vi "Organize Scouting Data.vi"() -> ()   [LabVIEW 2015]
uses:
  <vilib>/Utility/sysdir.llb/System Directory Type.ctl
panel:
  out "array averaged":string[][](array[string])
  out "array":string[][](array[string])
  out "reversed array":T1(array[cluster])
  in  "input cluster":T2
  out "output cluster":T2
  in  "Sort By":u16(ring) items=["Team Number", "Rating", "Number of High Goals", "Number of Low Goals"]
  in  "array type (2D Dbl)":string[][](array[string])
  # "Team Number"
  # "Lift Gate"
  # "Teeter Totter"
  # "Moat"
  # "Rampart"
  # "Drawbridge"
  # "Sally Port"
  # "Rock Wall"
  # "Rough Terrain"
  # "Low Bar"
  # "Auto High Goal"
  # "Auto Low Goal"
  # "Scale"
  # "High Goals"
  # "Low Goal"
  # "Autonomous"
  # "Up to Defense"
  # "Rating"
  # "Comment"
  # "Team Number"
  # "Lift Gate"
  # "Teeter Totter"
  # "Moat"
  # "Rampart"
  # "Drawbridge"
  # "Sally Port"
  # "Rock Wall"
  # "Rough Terrain"
  # "Low Bar"
  # "Auto High Goal"
  # "Auto Low Goal"
  # "Scale"
  # "High Goals"
  # "Low Goal"
  # "Autonomous"
  # "Up to Defense"
  # "Rating"
  # "Comment"
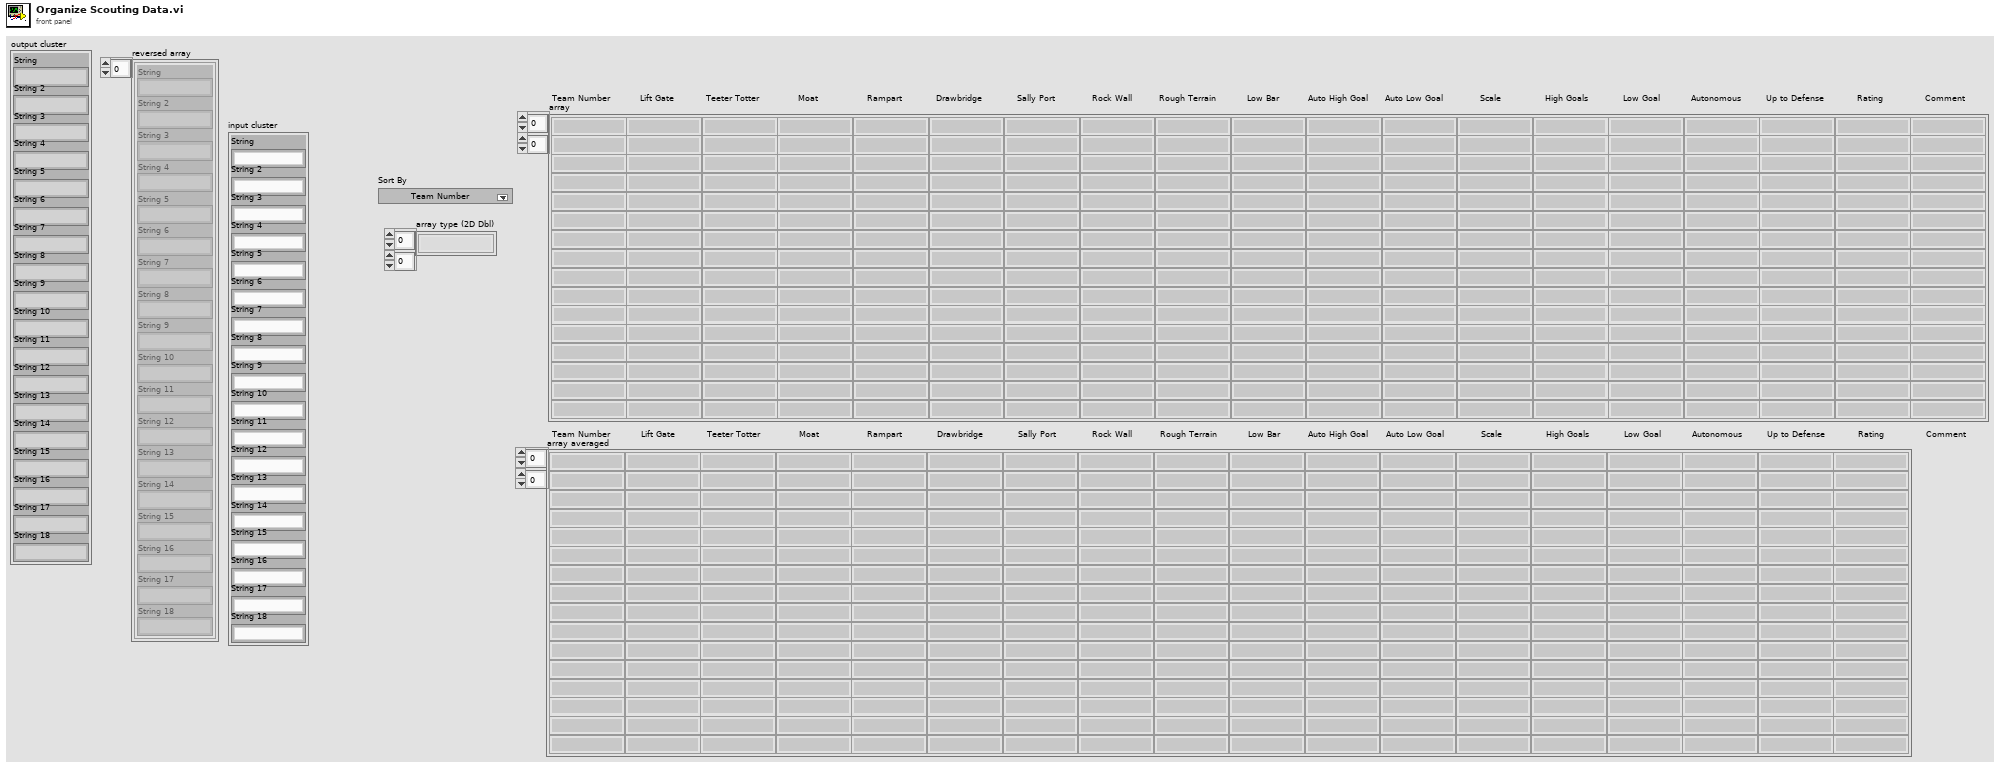
[diagram p1: front panel]
types:
  T1 = cluster{"String":string, "String 2":string, "String 3":string, "String 4":string, "String 5":string, "String 6":string, "String 7":string, "String 8":string, "String 9":string, "String 10":string, "String 11":string, "String 12":string, "String 13":string, "String 14":string, "String 15":string, "String 16":string, "String 17":string, "String 18":string}[]
  T2 = cluster{"String":string, "String 2":string, "String 3":string, "String 4":string, "String 5":string, "String 6":string, "String 7":string, "String 8":string, "String 9":string, "String 10":string, "String 11":string, "String 12":string, "String 13":string, "String 14":string, "String 15":string, "String 16":string, "String 17":string, "String 18":string}
  T3 = typedef "System Directory Type.ctl" = i32
  T4 = enum16{"open", "replace", "create", "open or create", "replace or create", "replace or create with confirmation"}
  T5 = cluster{string, string, string, string, string, string, string, string, string, string, string, string, string, string, string, string, string, string, string}[]
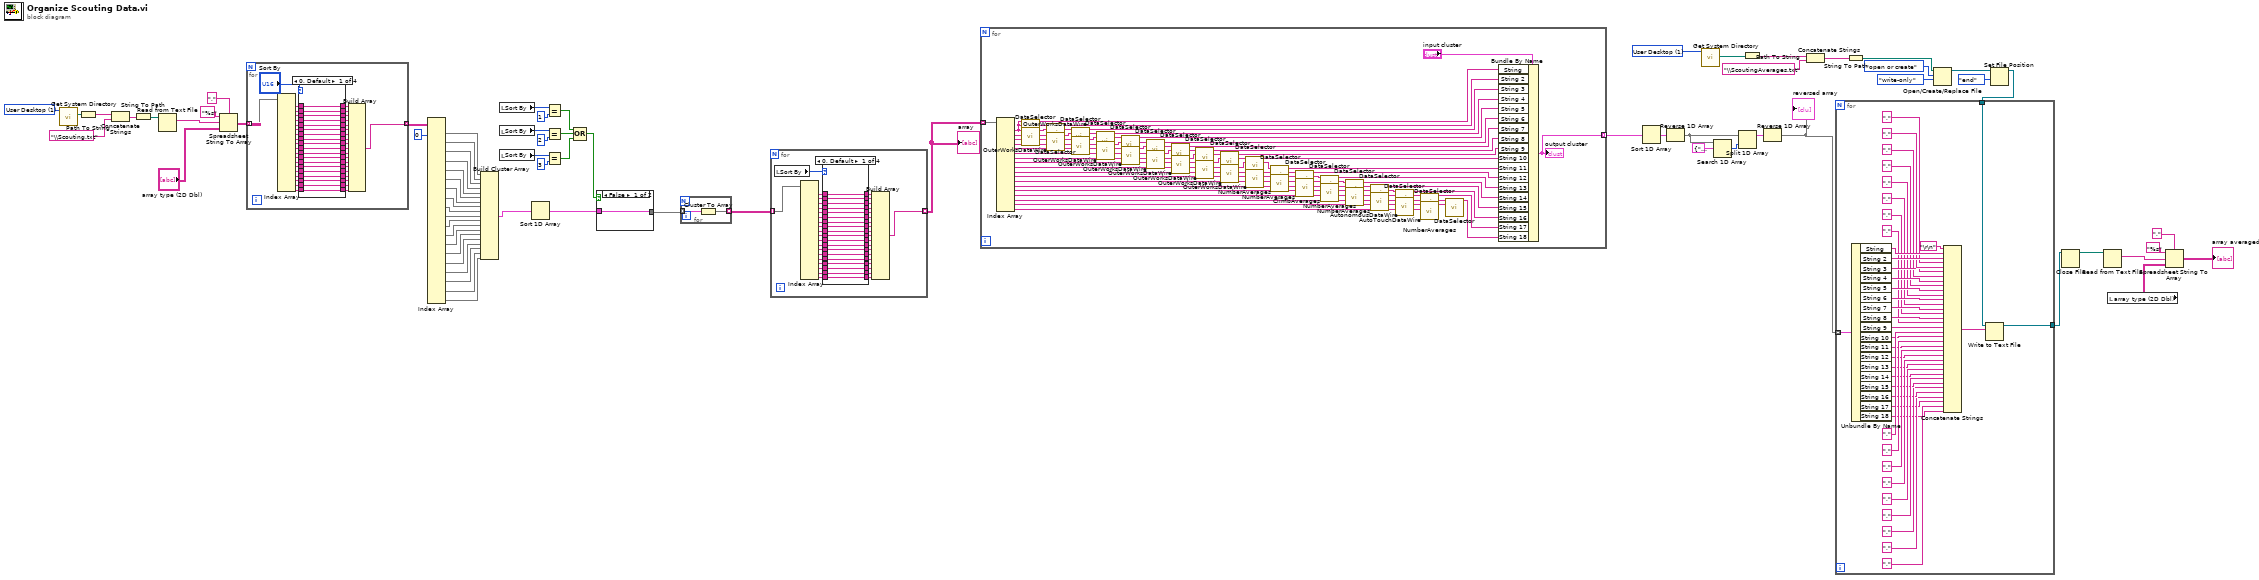
[diagram p0: block diagram]
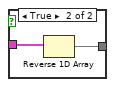
[diagram p5: hidden frame]
diagram:
  w15 = T3 1 items=["User Home"=0, "User Desktop"=1, "User Documents"=2, "User Application Data"=3, "User Preferences"=4, "User Temporary"=5, "Public Documents"=6, "Public Application Data"=7, "Public Preferences"=8, "Public Cache"=13, "System Core Libraries"=9, "System Installed Libraries"=10, "Application Files"=11, "Boot Volume Root"=12] ("system directory type")
  w68 = T3 1 items=["User Home"=0, "User Desktop"=1, "User Documents"=2, "User Application Data"=3, "User Preferences"=4, "User Temporary"=5, "Public Documents"=6, "Public Application Data"=7, "Public Preferences"=8, "Public Cache"=13, "System Core Libraries"=9, "System Installed Libraries"=10, "Application Files"=11, "Boot Volume Root"=12] ("system directory type")
  n1 = call <vilib>:"Get System Directory.vi"("system directory type"=w68) -> ("system directory"=w69:path)  [unwired: 10 in]
  n2 = Path To String(path=w69) -> (string=w70:string)
  n3 = Concatenate Strings(w70, "\\Scouting.txt" ("string")) -> (w72:string)
  n4 = String To Path(string=w72) -> (path=w67:path)
  n5 = Read from Text File(file (use dialog)=w67) -> (text=w64:string)  [unwired: 3 in, 3 out]
  n6 = Spreadsheet String To Array(delimiter (Tab)=",", format string="%s", spreadsheet string=w64, array type (2D Dbl)="array type (2D Dbl)") -> (array=w56:string[][])
  n7 = for {
    tunnel: w56 -> [w113] mode=indexing
    tunnel: [w76] -> w35 mode=indexing
    n8 = Index Array(array=w113) -> (element #1=w111:string, element #2=w109:string, element #3=w108:string, element #4=w105:string, element #5=w103:string, element #6=w101:string, element #7=w99:string, element #8=w97:string, element #9=w95:string, element #10=w93:string, element #11=w91:string, element #12=w89:string, element #13=w87:string, element #14=w85:string, element #15=w83:string, element #16=w81:string, element #17=w79:string, element #18=w77:string, element #19=w73:string)  [unwired: 19 in]
    n9 = case shown="0, Default" "Sort By" {
      tunnel: [w132 w150 w170 w172] -> w112
      tunnel: w111 -> [w132 w151 w169 w173]
      tunnel: [w131 w149 w168 w189] -> w110
      tunnel: w109 -> [w131 w149 w168 w189]
      tunnel: [w130 w148 w167 w188] -> w107
      tunnel: w108 -> [w130 w148 w167 w188]
      tunnel: [w129 w147 w166 w187] -> w106
      tunnel: w105 -> [w129 w147 w166 w187]
      tunnel: [w128 w146 w165 w186] -> w104
      tunnel: w103 -> [w128 w146 w165 w186]
      tunnel: [w127 w145 w164 w185] -> w102
      tunnel: w101 -> [w127 w145 w164 w185]
      tunnel: [w126 w144 w163 w184] -> w100
      tunnel: w99 -> [w126 w144 w163 w184]
      tunnel: [w125 w143 w162 w183] -> w98
      tunnel: w97 -> [w125 w143 w162 w183]
      tunnel: [w124 w142 w161 w182] -> w96
      tunnel: w95 -> [w124 w142 w161 w182]
      tunnel: [w123 w141 w160 w181] -> w94
      tunnel: w93 -> [w123 w141 w160 w181]
      tunnel: [w122 w140 w159 w180] -> w92
      tunnel: w91 -> [w122 w140 w159 w180]
      tunnel: [w121 w139 w158 w179] -> w90
      tunnel: w89 -> [w121 w139 w158 w179]
      tunnel: [w120 w138 w157 w178] -> w88
      tunnel: w87 -> [w120 w138 w157 w178]
      tunnel: [w119 w137 w169 w171] -> w86
      tunnel: w85 -> [w119 w137 w170 w171]
      tunnel: [w118 w136 w156 w173] -> w84
      tunnel: w83 -> [w118 w136 w156 w172]
      tunnel: [w117 w135 w155 w177] -> w82
      tunnel: w81 -> [w117 w135 w155 w177]
      tunnel: [w116 w134 w154 w176] -> w80
      tunnel: w79 -> [w116 w134 w154 w176]
      tunnel: [w115 w151 w153 w175] -> w78
      tunnel: w77 -> [w115 w150 w153 w175]
      tunnel: [w114 w133 w152 w174] -> w74
      tunnel: w73 -> [w114 w133 w152 w174]
      frame 0, Default {
      }
      frame 1 {
      }
      frame 2 {
      }
      frame 3 {
      }
    }
    n10 = Build Array(w112, w110, w107, w106, w104, w102, w100, w98, w96, w94, w92, w90, w88, w86, w84, w82, w80, w78, w74) -> (w76:string[])
  }
  n11 = Index Array(array=w35, index (col) #1=0 ("disabled index (col)")) -> (element #1=w55:string[], element #2=w54:string[], element #3=w53:string[], element #4=w52:string[], element #5=w51:string[], element #6=w50:string[], element #7=w49:string[], element #8=w48:string[], element #9=w47:string[], element #10=w46:string[], element #11=w45:string[], element #12=w44:string[], element #13=w43:string[], element #14=w42:string[], element #15=w41:string[], element #16=w40:string[], element #17=w39:string[], element #18=w38:string[], element #19=w36:string[])  [unwired: 37 in]
  n12 = Build Cluster Array ("Index & Bundle Cluster Array")(w55, w54, w53, w52, w51, w50, w49, w48, w47, w46, w45, w44, w43, w42, w41, w40, w39, w38, w36) -> (w37:T5)
  n13 = local read "Sort By"() -> (w32:u16)
  n14 = local read "Sort By"() -> (w29:u16)
  n15 = local read "Sort By"() -> (w28:u16)
  n16 = Sort 1D Array(array=w37) -> (sorted array=w34:T5)
  n17 = Equal?(x=w32, y=u16 1) -> (x = y?=w26:bool)
  n18 = Equal?(x=w29, y=u16 2) -> (x = y?=w25:bool)
  n19 = Equal?(x=w28, y=u16 3) -> (x = y?=w24:bool)
  n20 = Compound Arithmetic op=OR(w26, w25, w24) -> (w23:bool)
  n21 = case shown="False" w23 {
    tunnel: w34 -> [w190 w192]
    tunnel: [w190 w191] -> w33
    frame False {
    }
    frame True {
      n22 = Reverse 1D Array(array=w192) -> (reversed array=w191:T5)
    }
  }
  n23 = for {
    tunnel: w33 -> [w193] mode=indexing
    tunnel: [w194] -> w22 mode=indexing
    n24 = Cluster To Array(cluster=w193) -> (array=w194:string[])
  }
  n25 = for {
    tunnel: w22 -> [w235] mode=indexing
    tunnel: [w198] -> w20 mode=indexing
    n26 = local read "Sort By"() -> (w195:u16)
    n27 = Index Array(array=w235) -> (element #1=w233:string, element #2=w231:string, element #3=w230:string, element #4=w227:string, element #5=w225:string, element #6=w223:string, element #7=w221:string, element #8=w219:string, element #9=w217:string, element #10=w215:string, element #11=w213:string, element #12=w211:string, element #13=w209:string, element #14=w207:string, element #15=w205:string, element #16=w203:string, element #17=w201:string, element #18=w199:string, element #19=w196:string)  [unwired: 19 in]
    n28 = case shown="0, Default" w195 {
      tunnel: [w254 w272 w292 w294] -> w234
      tunnel: w233 -> [w254 w273 w291 w295]
      tunnel: [w253 w271 w290 w311] -> w232
      tunnel: w231 -> [w253 w271 w290 w311]
      tunnel: [w252 w270 w289 w310] -> w229
      tunnel: w230 -> [w252 w270 w289 w310]
      tunnel: [w251 w269 w288 w309] -> w228
      tunnel: w227 -> [w251 w269 w288 w309]
      tunnel: [w250 w268 w287 w308] -> w226
      tunnel: w225 -> [w250 w268 w287 w308]
      tunnel: [w249 w267 w286 w307] -> w224
      tunnel: w223 -> [w249 w267 w286 w307]
      tunnel: [w248 w266 w285 w306] -> w222
      tunnel: w221 -> [w248 w266 w285 w306]
      tunnel: [w247 w265 w284 w305] -> w220
      tunnel: w219 -> [w247 w265 w284 w305]
      tunnel: [w246 w264 w283 w304] -> w218
      tunnel: w217 -> [w246 w264 w283 w304]
      tunnel: [w245 w263 w282 w303] -> w216
      tunnel: w215 -> [w245 w263 w282 w303]
      tunnel: [w244 w262 w281 w302] -> w214
      tunnel: w213 -> [w244 w262 w281 w302]
      tunnel: [w243 w261 w280 w301] -> w212
      tunnel: w211 -> [w243 w261 w280 w301]
      tunnel: [w242 w260 w279 w300] -> w210
      tunnel: w209 -> [w242 w260 w279 w300]
      tunnel: [w241 w259 w291 w293] -> w208
      tunnel: w207 -> [w241 w259 w292 w293]
      tunnel: [w240 w258 w278 w295] -> w206
      tunnel: w205 -> [w240 w258 w278 w294]
      tunnel: [w239 w257 w277 w299] -> w204
      tunnel: w203 -> [w239 w257 w277 w299]
      tunnel: [w238 w256 w276 w298] -> w202
      tunnel: w201 -> [w238 w256 w276 w298]
      tunnel: [w237 w273 w275 w297] -> w200
      tunnel: w199 -> [w237 w272 w275 w297]
      tunnel: [w236 w255 w274 w296] -> w197
      tunnel: w196 -> [w236 w255 w274 w296]
      frame 0, Default {
      }
      frame 1 {
      }
      frame 2 {
      }
      frame 3 {
      }
    }
    n29 = Build Array(w234, w232, w229, w228, w226, w224, w222, w220, w218, w216, w214, w212, w210, w208, w206, w204, w202, w200, w197) -> (w198:string[])
  }
  "array" <- w20
  n30 = for {
    tunnel: w20 -> [w400] mode=indexing
    tunnel: [w399] -> w62 mode=indexing
    n31 = Index Array(array=w400) -> (element #1=w337:string, element #2=w336:string, element #3=w335:string, element #4=w334:string, element #5=w333:string, element #6=w332:string, element #7=w331:string, element #8=w330:string, element #9=w329:string, element #10=w328:string, element #11=w326:string, element #12=w324:string, element #13=w317:string, element #14=w316:string, element #15=w315:string, element #16=w314:string, element #17=w313:string, element #18=w312:string)  [unwired: 18 in]
    n32 = call "DataSelector.vi"("Number in"=w337, "String in"=w337) -> ("String out"=w394:string, "Number out"=w396:string)  [unwired: 12 in]
    n33 = call "OuterWorksDataWire.vi"("String in"=w336, "Number in"=w337) -> ("Number out"=w345:string, "String out"=w395:string)  [unwired: 8 in]
    n34 = call "DataSelector.vi"("Number in"=w396, "String in"=w395) -> ("String out"=w393:string, "Number out"=w392:string)  [unwired: 12 in]
    n35 = call "OuterWorksDataWire.vi"("String in"=w335, "Number in"=w345) -> ("Number out"=w344:string, "String out"=w391:string)  [unwired: 8 in]
    n36 = call "DataSelector.vi"("Number in"=w392, "String in"=w391) -> ("String out"=w397:string, "Number out"=w390:string)  [unwired: 12 in]
    n37 = call "OuterWorksDataWire.vi"("String in"=w334, "Number in"=w344) -> ("Number out"=w343:string, "String out"=w389:string)  [unwired: 8 in]
    n38 = call "DataSelector.vi"("Number in"=w390, "String in"=w389) -> ("String out"=w388:string, "Number out"=w387:string)  [unwired: 12 in]
    n39 = call "OuterWorksDataWire.vi"("String in"=w333, "Number in"=w343) -> ("Number out"=w342:string, "String out"=w386:string)  [unwired: 8 in]
    n40 = call "DataSelector.vi"("Number in"=w387, "String in"=w386) -> ("String out"=w385:string, "Number out"=w384:string)  [unwired: 12 in]
    n41 = call "OuterWorksDataWire.vi"("String in"=w332, "Number in"=w342) -> ("Number out"=w341:string, "String out"=w383:string)  [unwired: 8 in]
    n42 = call "DataSelector.vi"("Number in"=w384, "String in"=w383) -> ("String out"=w382:string, "Number out"=w381:string)  [unwired: 12 in]
    n43 = call "OuterWorksDataWire.vi"("String in"=w331, "Number in"=w341) -> ("Number out"=w340:string, "String out"=w380:string)  [unwired: 8 in]
    n44 = call "DataSelector.vi"("Number in"=w381, "String in"=w380) -> ("String out"=w379:string, "Number out"=w378:string)  [unwired: 12 in]
    n45 = call "OuterWorksDataWire.vi"("String in"=w330, "Number in"=w340) -> ("Number out"=w339:string, "String out"=w377:string)  [unwired: 8 in]
    n46 = call "DataSelector.vi"("Number in"=w378, "String in"=w377) -> ("String out"=w376:string, "Number out"=w375:string)  [unwired: 12 in]
    n47 = call "OuterWorksDataWire.vi"("String in"=w329, "Number in"=w339) -> ("Number out"=w338:string, "String out"=w374:string)  [unwired: 8 in]
    n48 = call "DataSelector.vi"("Number in"=w375, "String in"=w374) -> ("String out"=w373:string, "Number out"=w372:string)  [unwired: 12 in]
    n49 = call "OuterWorksDataWire.vi"("String in"=w328, "Number in"=w338) -> ("Number out"=w327:string, "String out"=w371:string)  [unwired: 8 in]
    n50 = call "DataSelector.vi"("Number in"=w372, "String in"=w371) -> ("String out"=w370:string, "Number out"=w369:string)  [unwired: 12 in]
    n51 = call "NumberAverages.vi"("Number in"=w327, "String in"=w326) -> ("String out"=w368:string, "Number out"=w325:string)  [unwired: 7 in]
    n52 = call "DataSelector.vi"("Number in"=w369, "String in"=w368) -> ("String out"=w367:string, "Number out"=w366:string)  [unwired: 12 in]
    n53 = call "NumberAverages.vi"("Number in"=w325, "String in"=w324) -> ("String out"=w365:string, "Number out"=w323:string)  [unwired: 7 in]
    n54 = call "DataSelector.vi"("Number in"=w366, "String in"=w365) -> ("String out"=w364:string, "Number out"=w363:string)  [unwired: 12 in]
    n55 = call "ClimbAverages.vi"("Number in"=w323, "String in"=w317) -> ("String out"=w362:string, "Number out"=w322:string)  [unwired: 7 in]
    n56 = call "DataSelector.vi"("Number in"=w363, "String in"=w362) -> ("String out"=w361:string, "Number out"=w360:string)  [unwired: 12 in]
    n57 = call "NumberAverages.vi"("Number in"=w322, "String in"=w316) -> ("String out"=w359:string, "Number out"=w321:string)  [unwired: 7 in]
    n58 = call "DataSelector.vi"("Number in"=w360, "String in"=w359) -> ("String out"=w358:string, "Number out"=w357:string)  [unwired: 12 in]
    n59 = call "NumberAverages.vi"("Number in"=w321, "String in"=w315) -> ("String out"=w356:string, "Number out"=w320:string)  [unwired: 7 in]
    n60 = call "DataSelector.vi"("Number in"=w357, "String in"=w356) -> ("String out"=w355:string, "Number out"=w354:string)  [unwired: 12 in]
    n61 = call "AutonomousDataWire.vi"("String in"=w314, "Number in"=w320) -> ("String out"=w319:string, "Number out"=w353:string)  [unwired: 8 in]
    n62 = call "DataSelector.vi"("Number in"=w354, "String in"=w353) -> ("String out"=w352:string, "Number out"=w351:string)  [unwired: 12 in]
    n63 = call "AutoTouchDataWire.vi"("String in"=w313, "Number in"=w319) -> ("Number out"=w318:string, "String out"=w350:string)  [unwired: 8 in]
    n64 = call "DataSelector.vi"("Number in"=w351, "String in"=w350) -> ("String out"=w349:string, "Number out"=w348:string)  [unwired: 12 in]
    n65 = call "NumberAverages.vi"("Number in"=w318, "String in"=w312) -> ("String out"=w346:string)  [unwired: 7 in, 1 out]
    n66 = call "DataSelector.vi"("Number in"=w348, "String in"=w346) -> ("String out"=w347:string)  [unwired: 12 in, 1 out]
    n67 = Bundle By Name(cluster="input cluster", "String"=w394, "String 2"=w393, "String 3"=w397, "String 4"=w388, "String 5"=w385, "String 6"=w382, "String 7"=w379, "String 8"=w376, "String 9"=w373, "String 10"=w370, "String 11"=w367, "String 12"=w364, "String 13"=w361, "String 14"=w358, "String 15"=w355, "String 16"=w352, "String 17"=w349, "String 18"=w347) -> (w399:T2)
    "output cluster" <- w399
  }
  n68 = Sort 1D Array(array=w62) -> (sorted array=w61:T1)
  n69 = Reverse 1D Array(array=w61) -> (reversed array=w58:T1)
  n70 = call <vilib>:"Get System Directory.vi"("system directory type"=w15) -> ("system directory"=w14:path)  [unwired: 10 in]
  n71 = Search 1D Array(1D array=w58, element=T2 {"String"="", "String 2"="", "String 3"="", "String 4"="", "String 5"="", "String 6"="", "String 7"="", "String 8"="", "String 9"="", "String 10"="", "String 11"="", "String 12"="", "String 13"="", "String 14"="", "String 15"="", "String 16"="", "String 17"="", "String 18"=""}) -> (index of element=w59:i32)  [unwired: 1 in]
  n72 = Split 1D Array(array=w58, index=w59) -> (first subarray=w57:T1)  [unwired: 1 out]
  n73 = Path To String(path=w14) -> (string=w13:string)
  n74 = Reverse 1D Array(array=w57) -> (reversed array=w9:T1)
  "reversed array" <- w9
  n75 = Concatenate Strings(w13, "\\ScoutingAverages.txt" ("string")) -> (w11:string)
  n76 = String To Path(string=w11) -> (path=w10:path)
  n77 = Open/Create/Replace File(file path (use dialog)=w10, operation (0:open)=T4."open or create", access (0:read/write)=enum16{"read/write", "read-only", "write-only"}."write-only") -> (refnum out=w17:refnum<file>)  [unwired: 3 in, 2 out]
  n78 = Set File Position(refnum=w17, from (0:start)=enum16{"start", "end", "current"}."end") -> (refnum out=w8:refnum<file>)  [unwired: 2 in, 1 out]
  n79 = for {
    tunnel: w9 -> [w440] mode=indexing
    tunnel: w8 -> [w402]
    tunnel: [w401] -> w7
    n80 = Unbundle By Name(w440) -> ("String"=w439:string, "String 2"=w437:string, "String 3"=w435:string, "String 4"=w433:string, "String 5"=w431:string, "String 6"=w429:string, "String 7"=w427:string, "String 8"=w425:string, "String 9"=w423:string, "String 10"=w421:string, "String 11"=w419:string, "String 12"=w417:string, "String 13"=w415:string, "String 14"=w413:string, "String 15"=w411:string, "String 16"=w409:string, "String 17"=w407:string, "String 18"=w405:string)
    n81 = Concatenate Strings("\r\n", w439, "," ("string"), w437, "," ("string"), w435, "," ("string"), w433, "," ("string"), w431, "," ("string"), w429, "," ("string"), w427, "," ("string"), w425, "," ("string"), w423, "," ("string"), w421, "," ("string"), w419, "," ("string"), w417, "," ("string"), w415, "," ("string"), w413, "," ("string"), w411, "," ("string"), w409, "," ("string"), w407, "," ("string"), w405) -> (w403:string)
    n82 = Write to Text File(file (use dialog)=w402, text=w403) -> (refnum out=w401:refnum<file>)  [unwired: 2 in, 2 out]
  }
  n83 = Close File(refnum=w7) -> (path=w3:path)  [unwired: 1 in, 1 out]
  n84 = Read from Text File(file (use dialog)=w3) -> (text=w4:string)  [unwired: 3 in, 3 out]
  n85 = local read "array type (2D Dbl)"() -> (w2:string[][])
  n86 = Spreadsheet String To Array(delimiter (Tab)=",", format string="%s", spreadsheet string=w4, array type (2D Dbl)=w2) -> (array=→"array averaged":string[][])
